vi "GeneralShotParameters.vi"(4 "Shot Quality":string(combo), 6 "System Message":string, 7 "TreeNode Path In":string, 8 "Error In":errorcluster, 9 "User Shot Notes":string, 10 "Current shot":i32, 11 "Tree DVR Input":refnum<data-value>) -> (0 "Error Out":errorcluster)   [LabVIEW 2013]
uses:
  <vilib>/MDSplus/Classes/Tree_Class/Tree.lvclass
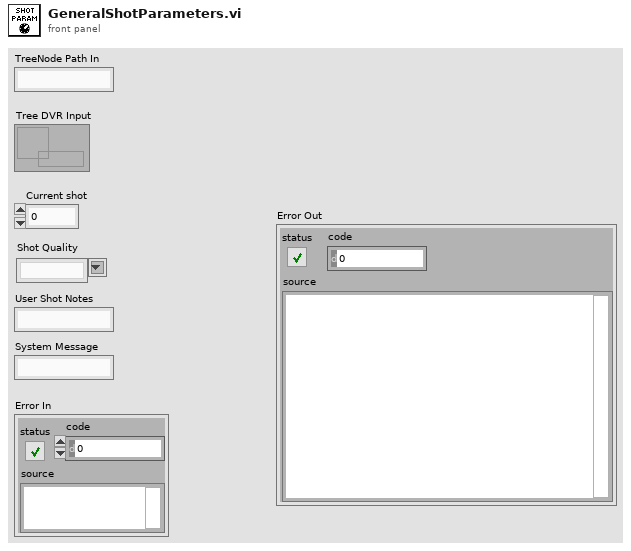
[diagram p1: front panel]
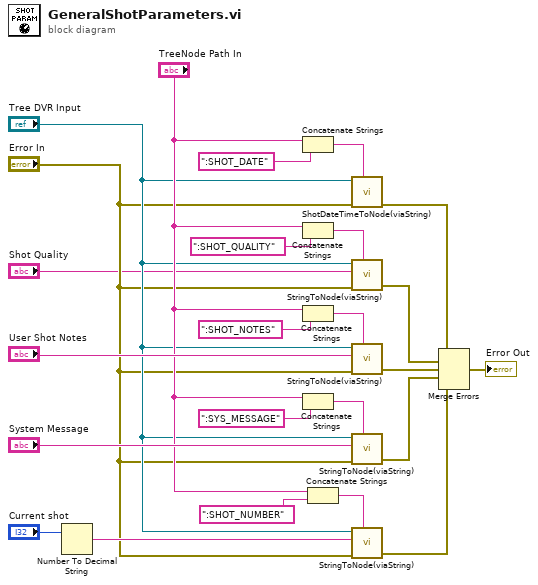
[diagram p0: block diagram]
diagram:
  n1 = Number To Decimal String(number="Current shot") -> (decimal integer string=w12:string)  [unwired: 1 in]
  n2 = Concatenate Strings("TreeNode Path In", ":SHOT_DATE") -> (w15:string)
  n3 = Concatenate Strings("TreeNode Path In", ":SHOT_QUALITY" ("NodePath")) -> (w9:string)
  n4 = Concatenate Strings("TreeNode Path In", ":SHOT_NOTES" ("NodePath")) -> (w17:string)
  n5 = Concatenate Strings("TreeNode Path In", ":SYS_MESSAGE" ("NodePath")) -> (w20:string)
  n6 = Concatenate Strings("TreeNode Path In", ":SHOT_NUMBER" ("string")) -> (w22:string)
  n7 = call "ShotDateTimeToNode(viaString).vi"("DateTime Path"=w15, "error in"="Error In", "Tree DVR in"="Tree DVR Input") -> ("error out"=w5:errorcluster)  [unwired: 8 in]
  n8 = call "StringToNode(viaString).vi"("Tree DVR in"="Tree DVR Input", "String value in"="Shot Quality", "error in (no error)"="Error In", "NodePath"=w9) -> ("error out"=w4:errorcluster)  [unwired: 1 in, 2 out]
  n9 = call "StringToNode(viaString).vi"("Tree DVR in"="Tree DVR Input", "String value in"="User Shot Notes", "error in (no error)"="Error In", "NodePath"=w17) -> ("error out"=w3:errorcluster)  [unwired: 1 in, 2 out]
  n10 = call "StringToNode(viaString).vi"("Tree DVR in"="Tree DVR Input", "String value in"="System Message", "error in (no error)"="Error In", "NodePath"=w20) -> ("error out"=w2:errorcluster)  [unwired: 1 in, 2 out]
  n11 = call "StringToNode(viaString).vi"("Tree DVR in"="Tree DVR Input", "String value in"=w12, "error in (no error)"="Error In", "NodePath"=w22) -> ("error out"=w1:errorcluster)  [unwired: 1 in, 2 out]
  n12 = Merge Errors(w5, w4, w3, w2, w1) -> (→"Error Out":errorcluster)
